vi "Verify Errors.vi"(6 "Top Ref":refnum<vi>, 8 "STOP? In":bool, 11 "error in":errorcluster) -> (0 "STOP? Out":bool, 3 "error out":errorcluster)   [LabVIEW 2024, in "User Interface.lvlib"]
uses:
  User Interface.lvlib
  Error Handler/Error Handler.lvlib
  UI Queue - Get.vi
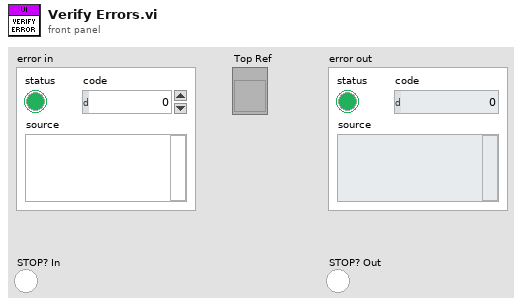
[diagram p1: front panel]
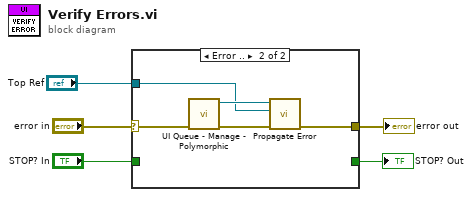
[diagram p0: block diagram]
diagram:
  n1 = case shown="Error .." "error in" {
    selector: "error in" -> [w7 w9]
    tunnel: [w7 w10] -> w4
    tunnel: "STOP? In" -> [w6 _]
    tunnel: [w6 _] -> w5
    tunnel: "Top Ref" -> [_ w8]
    frame No Error {
    }
    frame Error {
      n2 = call-poly "UI Queue - Manage - Polymorphic.vi"("error in"=w9) -> ("error out"=w11:errorcluster, "queue out"=w12:refnum<queue>)  [unwired: 9 in]
      n3 = call "Propagate Error.vi"("error in"=w11, "Issued VI"=w8, "queue out"=w12) -> ("error out"=w10:errorcluster)  [unwired: 8 in]
    }
  }
  "STOP? Out" <- w5
  "error out" <- w4
